vi "SendTcpMessage.vi"(6 "timeout (5 sec)":i32=5000, 7 "file":bool, 8 "error in (no error)":errorcluster, 10 "message":T1, 11 "connection ID in":T4) -> (0 "error out":errorcluster, 1 "error57":bool, 3 "connection ID out":T4)   [LabVIEW 2017]
uses:
  <vilib>/addons/InsightCM/MessageBus/TcpApi/controls/TcpMessageReference.ctl
  <vilib>/addons/InsightCM/MessageBus/Base/controls/Message.ctl
  <vilib>/addons/InsightCM/MessageBus/Base/controls/MessageHeader.ctl
  <vilib>/addons/InsightCM/MessageBus/Base/controls/KeyValuePair.ctl
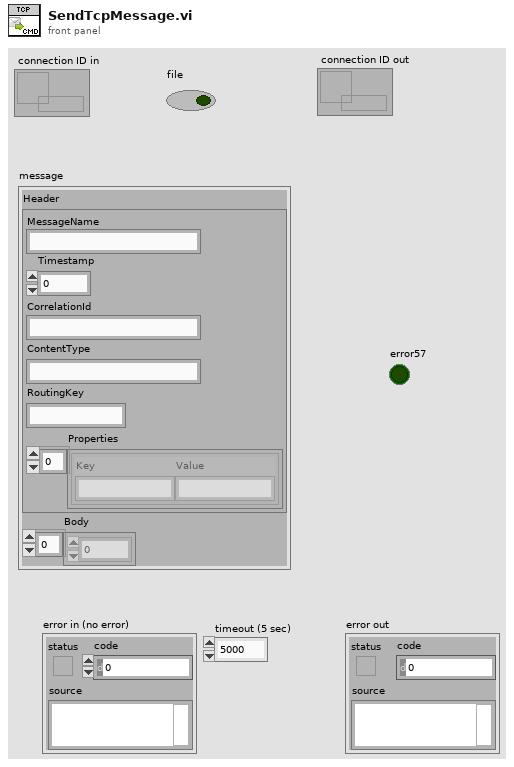
[diagram p1: front panel]
types:
  T1 = typedef "Message.ctl" = cluster{"Header":T2, "Body":u8[]}
  T2 = typedef "MessageHeader.ctl" = cluster{"MessageName":string, "Timestamp":i64, "CorrelationId":string, "ContentType":string, "RoutingKey":string, "Properties":T3[]}
  T3 = typedef "KeyValuePair.ctl" = cluster{"Key":string, "Value":string}
  T4 = typedef "TcpMessageReference.ctl" = refnum<data-value>
  T5 = cluster{"DeviceId":string, "CmdStream":refnum<k5>, "FileStream":refnum<k5>}
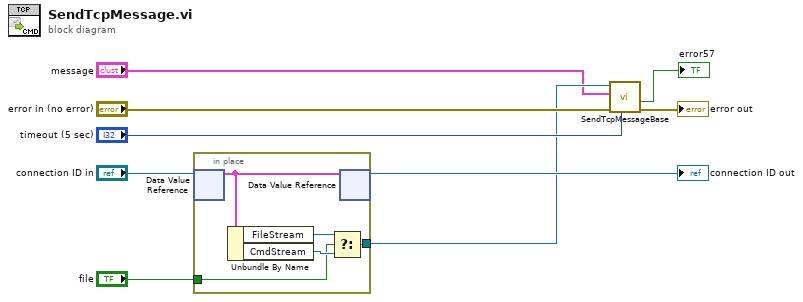
[diagram p0: block diagram]
diagram:
  n1 = in-place {
    in-place-border: "file" -> [w11]
    in-place-border: [w10] -> w3
    n2 = in-place-dvr #1("connection ID in") -> (w14:T5)  [unwired: 1 out]
    n3 = Unbundle By Name(w14) -> ("FileStream"=w13:refnum<k5>, "CmdStream"=w12:refnum<k5>)
    n4 = Select(t=w13, s=w11, f=w12) -> (s? t:f=w10:refnum<k5>)
    n5 = in-place-dvr #1(w14) -> (→"connection ID out":T4)  [unwired: 1 out]
  }
  n6 = call <vilib>:"SendTcpMessageBase.vi"("timeout (5 sec)"="timeout (5 sec)", "error in (no error)"="error in (no error)", "Message"="message", "tcp in"=w3) -> ("error out"=→"error out":errorcluster, "error57"=→"error57":bool)  [unwired: 5 in, 1 out]
